vi "Init Gyro.vi"(8 "error in (no error)":errorcluster) -> (0 "error out":errorcluster, 1 "Gyro Bias":cluster{"X":dbl, "Y":dbl, "Z":dbl}, 3 "I2C Ref Out":T1)   [LabVIEW 2018]
uses:
  <vilib>/myRIO/Instrument Drivers/Onboard IO/I2C/typedefs/I2C Reference.ctl
  <vilib>/myRIO/Common/Instrument Driver Framework/Utilities/typedefs/myRIO Generic Hardware Reference.ctl
  <vilib>/myRIO/Common/Instrument Driver Framework/Utilities/typedefs/Hardware Version Enum.ctl
  <vilib>/myRIO/Common/Instrument Driver Framework/Utilities/typedefs/myRIO v1.0 Reference.ctl
  <vilib>/myRIO/Common/Instrument Driver Framework/Utilities/typedefs/Generic FPGA Reference.ctl
  <vilib>/myRIO/Common/Instrument Driver Framework/myRIO v1.0/I2C/typedefs/I2C Channels Enum.ctl
  <vilib>/myRIO/Instrument Drivers/Onboard IO/I2C/typedefs/I2C Configuration.ctl
  <vilib>/myRIO/Instrument Drivers/Onboard IO/I2C/typedefs/I2C Transfer Rate.ctl
  lib/MPU6050 Private class data.vi
  <vilib>/myRIO/Instrument Drivers/Onboard IO/I2C/I2C.lvlib
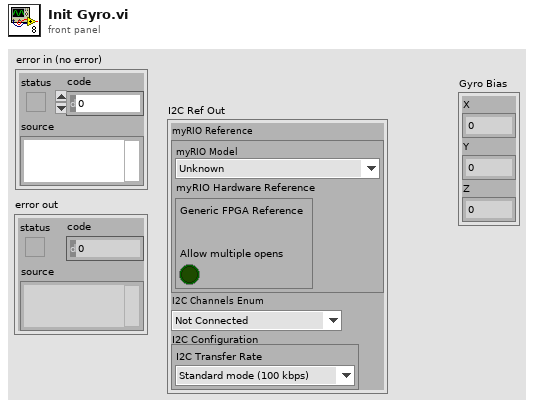
[diagram p1: front panel]
types:
  T1 = typedef "I2C.lvlib/I2C Reference.ctl" = cluster{"myRIO Reference":T2, "I2C Channels Enum":T6, "I2C Configuration":T7}
  T2 = typedef "myRIO Generic Hardware Reference.ctl" = cluster{"myRIO Model":T3, "myRIO Hardware Reference":T4}
  T3 = typedef "Hardware Version Enum.ctl" = enum16{"Unknown", "myRIO-1900", "myRIO-1950", "roboRIO", "NI ELVIS RIO CM", "ELVIS III"}
  T4 = typedef "myRIO v1.0 Reference.ctl" = cluster{"Generic FPGA Reference":T5, "Allow multiple opens":bool}
  T5 = typedef "Generic FPGA Reference.ctl" = refnum<k20>
  T6 = typedef "I2C Channels Enum.ctl" = enum16{"Not Connected", "A/I2C", "B/I2C", "I2C/I2C"}
  T7 = typedef "I2C.lvlib/I2C Configuration.ctl" = cluster{"I2C Transfer Rate":T8}
  T8 = typedef "I2C.lvlib/I2C Transfer Rate.ctl" = enum16{"Standard mode (100 kbps)", "Fast mode (400 kbps)"}
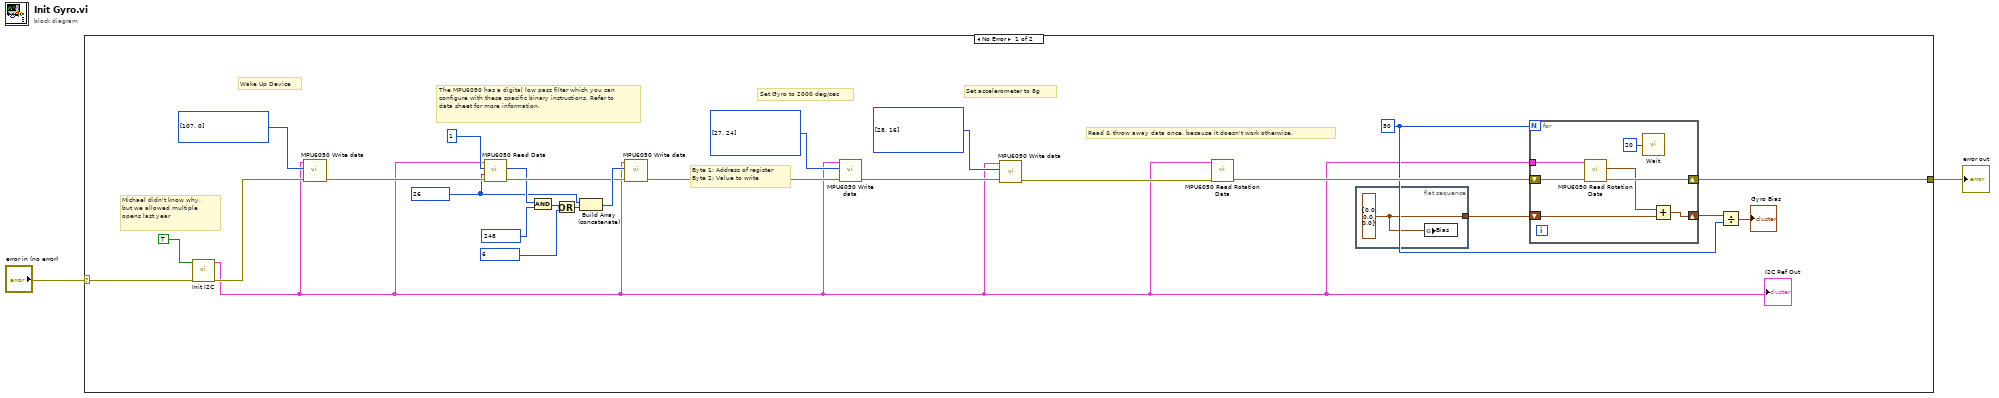
[diagram p0: block diagram]
diagram:
  n1 = case shown="No Error" "error in (no error)" {
    selector: "error in (no error)" -> [w28 w37]
    tunnel: [w27 w37] -> w1
    frame No Error {
      w12 = u8 26
      w24 = 50
      # "Byte 1: Address of register\nByte 2: Value to write"
      # "Set accelerometer to 8g"
      # "Michael didn't know why, but we allowed multiple opens last year"
      # "Wake Up Device"
      # "The MPU6050 has a digital low pass filter which you can configure with these specific binary instructions. Refer to data sheet for more information."
      # "Set Gyro to 2000 deg/sec"
      # "Read & throw away data once, because it doesn't work otherwise."
      n2 = call "Init I2C.vi"("error in"=w28, "Allow multiple opens?"=TRUE) -> ("error out"=w10:errorcluster, "I2C Ref Out"=w3:T1)  [unwired: 8 in]
      "I2C Ref Out" <- w3
      n3 = call "MPU6050 Write data.vi"("I2C Ref In"=w3, "Bytes to Write"=u8[] [107, 0], "error in (no error)"=w10) -> ("error out"=w15:errorcluster)  [unwired: 7 in]
      n4 = call "MPU6050 Read Data.vi"("error in (no error)"=w15, "Start Address"=w12, "Data Length"=u8 1, "I2C Ref In"=w3) -> ("error out"=w16:errorcluster, "Data read"=w13:u8[])  [unwired: 6 in]
      n5 = And(x=w13, y=u8 248) -> (x .and. y?=w19:u8[])
      n6 = Or(x=w19, y=u8 6) -> (x .or. y?=w20:u8[])
      n7 = Build Array (concatenate)(w12, w20) -> (w17:u8[])
      n8 = call "MPU6050 Write data.vi"("I2C Ref In"=w3, "Bytes to Write"=w17, "error in (no error)"=w16) -> ("error out"=w23:errorcluster)  [unwired: 7 in]
      n9 = call "MPU6050 Write data.vi"("I2C Ref In"=w3, "Bytes to Write"=u8[] [27, 24], "error in (no error)"=w23) -> ("error out"=w6:errorcluster)  [unwired: 7 in]
      n10 = call "MPU6050 Write data.vi"("I2C Ref In"=w3, "Bytes to Write"=u8[] [28, 16], "error in (no error)"=w6) -> ("error out"=w5:errorcluster)  [unwired: 7 in]
      n11 = call "MPU6050 Read Rotation Data.vi"("error in (no error)"=w5, "I2C Ref In"=w3) -> ("error out"=w26:errorcluster)  [unwired: 7 in, 2 out]
      n12 = flat-sequence {
        tunnel: [w29] -> w8
        frame #0 {
          w29 = cluster{"X":dbl, "Y":dbl, "Z":dbl} {"X"=0.0, "Y"=0.0, "Z"=0.0} ("Gyro Data")
          n13 = global write "MPU6050 Private class data.vi" "Bias"(w29) -> ()
        }
      }
      n14 = for {
        N: w24 -> [_]
        shift-right: [w35] -> w27
        shift-left: w26 -> [w36]
        shift-right: [w34] -> w25
        shift-left: w8 -> [w32]
        tunnel: w3 -> [w30]
        n15 = call "MPU6050 Read Rotation Data.vi"("error in (no error)"=w36, "I2C Ref In"=w30) -> ("error out"=w35:errorcluster, "rad/s"=w33:cluster{"X":dbl, "Y":dbl, "Z":dbl})  [unwired: 7 in, 1 out]
        n16 = call "Wait"("Count(mSec)"=u32 20 ("Count(uSec)")) -> ()  [unwired: 1 out]
        n17 = Add(x=w33, y=w32) -> (x+y=w34:cluster{"X":dbl, "Y":dbl, "Z":dbl})
      }
      n18 = Divide(x=w25, y=w24) -> (x/y=→"Gyro Bias":cluster{"X":dbl, "Y":dbl, "Z":dbl})
    }
    frame Error {
    }
  }
  "error out" <- w1
